vi "PicoErrorString.vi"(4 "error in":errorcluster) -> (0 "[user-defined descriptions]":string[](array[string]), 1 "String":string, 3 "[user-defined codes]":u32[](array[numeric])=[5001, 5002, 5003, 5004, 5005, 5006, 5007, 5008, 5009, 5010, 5011, 5012, 5013, 5014, 5015, 5016, 5017, 5018, 5019, 5020, 5021, 5022, 5023, 5024, 5025, 5026, 5027, 5028, 5029, 5030, 5031, 5032, 5033, 5034, 5035, 5036, 5037, 5038, 5039, 5040, 5041, 5042, 5043, 5044, 5045, 5046, 5047, 5048, 5049, 5050, 5051, 5052, 5053, 5054, 5055, 5056, 5057, 5058, 5059, 5060, 5061, 5063, 5064, 5065, 5066, 5067, 5068, 5069, 5070, 5071, 5072, 5073, 5074, 5075, 5076, 5077, 5078, 5079, 5080, 5081, 5082, 5083, 5084, 5086, 5087, 5088, 5089, 5259, 5260, 5261, 5262, 5263, 5264, 5265, 5266, 5267, 5268, 5269, 5270, 5271, 5272, 5273, 5274, 5275, 5276, 5277, 5278, 5279, 5280, 5281, 5282, 5283, 5284, 5285, 5286, 5287, 5288, 5289, 5290, 5291, 5292, 5293, 5294, 5295, 5296, 5297, 5298, 5299, 5300, 5301, 5302, 5303, 5304, 5305, 5306, 5307, 5308, 5309, 5310, 5311, 5312, 5313, 5314, 5315, 5316, 5317, 5318, 5319, 5320, 5321, 5090, 5091, 5092, 5093, 5094, 5095, 5096, 5097, 5322, 5323, 5324, 5325, 5326, 5327, 5328, 5329, 5330, 5331, 5332, 5333, 5334, 5335, 5336, 5337, 5338, 5339, 5340, 5341, 5342, 5343, 16782216, 268440456, 268440457, 268440458, 268440459, 268440460, 268440461, 268440462, 268440463, 268440464, 285217672])   [LabVIEW 2020]
doc: "This VI takes an error cluster and if an error has occurred, displays a message box indicating the source of the error and the status code returned by the driver."
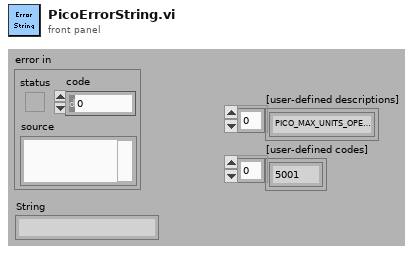
[diagram p1: front panel]
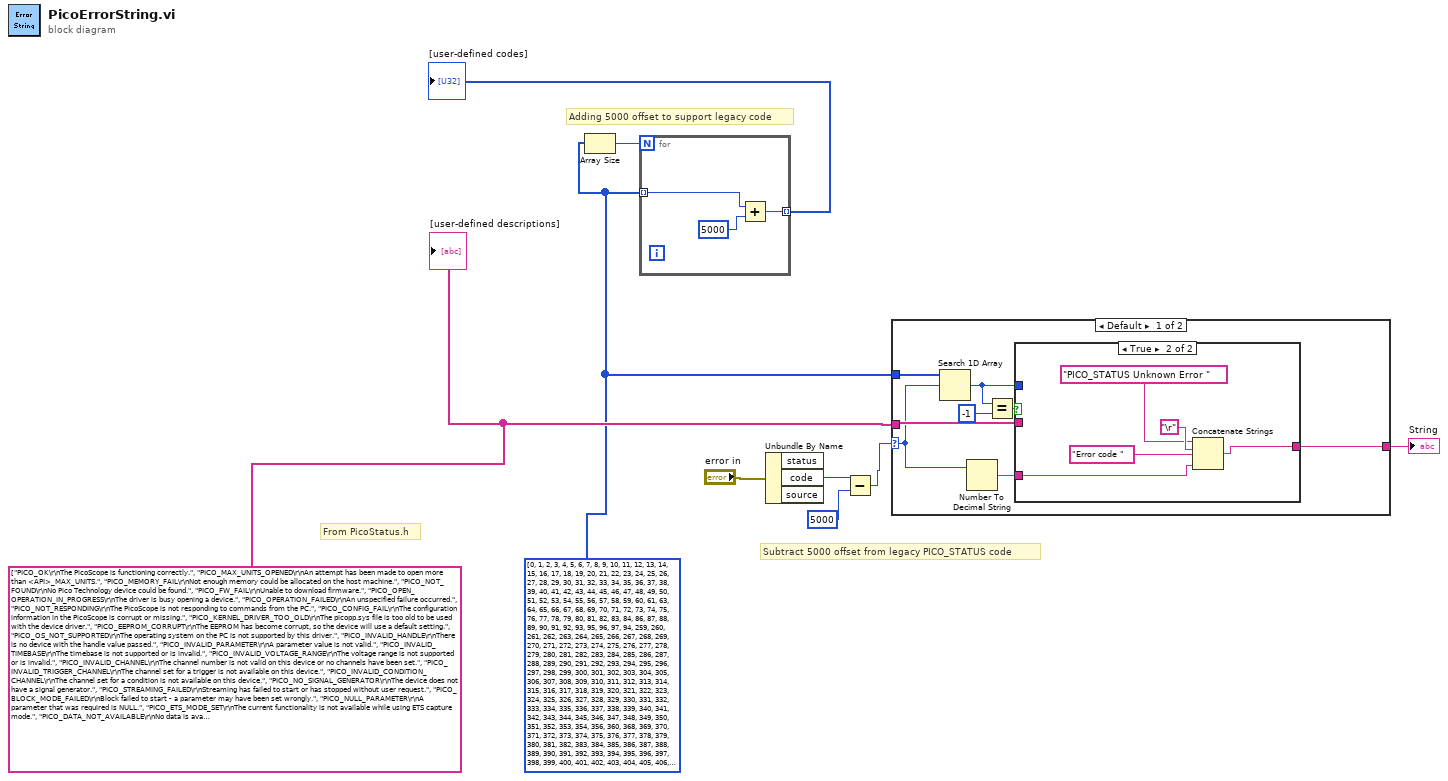
[diagram p0: block diagram]
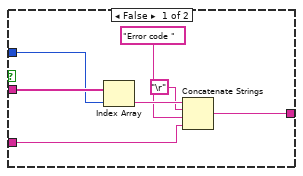
[diagram p2: hidden frame]
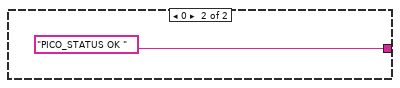
[diagram p3: hidden frame]
diagram:
  w1 = u32[] [0, 1, 2, 3, 4, 5, 6, 7, 8, 9, 10, 11, 12, 13, 14, 15, 16, 17, 18, 19, 20, 21, 22, 23, 24, 25, 26, 27, 28, 29, 30, 31, 32, 33, 34, 35, 36, 37, 38, 39, 40, 41, 42, 43, 44, 45, 46, 47, 48, 49, 50, 51, 52, 53, 54, 55, 56, 57, 58, 59, 60, 61, 63, 64, 65, 66, 67, 68, 69, 70, 71, 72, 73, 74, 75, 76, 77, 78, 79, 80, 81, 82, 83, 84, 86, 87, 88, 89, 90, 91, 92, 93, 95, 96, 97, 94, 259, 260, 261, 262, 263, 264, 265, 266, 267, 268, 269, 270, 271, 272, 273, 274, 275, 276, 277, 278, 279, 280, 281, 282, 283, 284, 285, 286, 287, 288, 289, 290, 291, 292, 293, 294, 295, 296, 297, 298, 299, 300, 301, 302, 303, 304, 305, 306, 307, 308, 309, 310, 311, 312, 313, 314, 315, 316, 317, 318, 319, 320, 321, 322, 323, 324, 325, 326, 327, 328, 329, 330, 331, 332, 333, 334, 335, 336, 337, 338, 339, 340, 341, 342, 343, 344, 345, 346, 347, 348, 349, 350, 351, 352, 353, 354, 356, 360, 368, 369, 370, 371, 372, 373, 374, 375, 376, 377, 378, 379, 380, 381, 382, 383, 384, 385, 386, 387, 388, 389, 390, 391, 392, 393, 394, 395, 396, 397, 398, 399, 400, 401, 402, 403, 404, 405, 406, 407, 408, 409, 410, 411, 412, 413, 512, 513, 514, 515, 516, 521, 522, 523, 524, 525, 526, 528, 529, 530, 531, 768, 769, 770, 4096, 4097, 8192, 8193, 8194, 8195, 8196, 8197, 8198, 8199, 8200, 8203, 8204, 8205, 8206, 8207, 8208, 8209, 8210, 8211, 8212, 8213, 8214, 8215, 8216, 8217, 12288, 12289, 12290, 12291, 12292, 12293, 12294, 12295, 12296, 12297, 12298, 12299, 16384, 20480, 20481, 20482, 20483, 20484, 20485, 20496, 24576, 24577, 24578, 28672, 28673, 28674, 16777216, 33554433, 33554434, 33554436, 33554440, 33554688, 35651584, 35651585, 35651586, 35651587, 35651588, 35651589, 35651590, 35651591, 50331664, 50331665, 50331666, 50331667, 50331668, 50331669, 50331680, 50331681, 50331682, 50331683, 50331684, 50331685, 50331686, 50331687, 50331696, 50331697, 50331698, 50331699, 50331700, 50331701, 50331702, 50331703, 50331704, 50331705, 50331712, 50335744, 50343937, 50343938, 50343939, 50345984, 50348032, 50348033, 50348034, 50348035, 50348036, 50348037, 50348038, 50348039, 50348040, 50348041, 50364416, 50364417, 50339840, 268435456, 268435457, 268435458, 268435459, 268435460, 268435461, 268435462, 268435463, 268435464, 268435472, 285212672, 536870912, 536870913, 536870914, 536870915, 536870916, 536870917, 536870918, 536870919, 536870920, 536870921] ("PICO_STATUS codes")
  w2 = string[] ["PICO_OK\r\nThe PicoScope is functioning correctly.", "PICO_MAX_UNITS_OPENED\r\nAn attempt has been made to open more than <API>_MAX_UNITS.", "PICO_MEMORY_FAIL\r\nNot enough memory could be allocated on the host machine.", "PICO_NOT_FOUND\r\nNo Pico Technology device could be found.", "PICO_FW_FAIL\r\nUnable to download firmware.", "PICO_OPEN_OPERATION_IN_PROGRESS\r\nThe driver is busy opening a device.", "PICO_OPERATION_FAILED\r\nAn unspecified failure occurred.", "PICO_NOT_RESPONDING\r\nThe PicoScope is not responding to commands from the PC.", "PICO_CONFIG_FAIL\r\nThe configuration information in the PicoScope is corrupt or missing.", "PICO_KERNEL_DRIVER_TOO_OLD\r\nThe picopp.sys file is too old to be used with the device driver.", "PICO_EEPROM_CORRUPT\r\nThe EEPROM has become corrupt, so the device will use a default setting.", "PICO_OS_NOT_SUPPORTED\r\nThe operating system on the PC is not supported by this driver.", "PICO_INVALID_HANDLE\r\nThere is no device with the handle value passed.", "PICO_INVALID_PARAMETER\r\nA parameter value is not valid.", "PICO_INVALID_TIMEBASE\r\nThe timebase is not supported or is invalid.", "PICO_INVALID_VOLTAGE_RANGE\r\nThe voltage range is not supported or is invalid.", "PICO_INVALID_CHANNEL\r\nThe channel number is not valid on this device or no channels have been set.", "PICO_INVALID_TRIGGER_CHANNEL\r\nThe channel set for a trigger is not available on this device.", "PICO_INVALID_CONDITION_CHANNEL\r\nThe channel set for a condition is not available on this device.", "PICO_NO_SIGNAL_GENERATOR\r\nThe device does not have a signal generator.", "PICO_STREAMING_FAILED\r\nStreaming has failed to start or has stopped without user request.", "PICO_BLOCK_MODE_FAILED\r\nBlock failed to start - a parameter may have been set wrongly.", "PICO_NULL_PARAMETER\r\nA parameter that was required is NULL.", "PICO_ETS_MODE_SET\r\nThe current functionality is not available while using ETS capture mode.", "PICO_DATA_NOT_AVAILABLE\r\nNo data is available from a run block call.", "PICO_STRING_BUFFER_TO_SMALL\r\nThe buffer passed for the information was too small.", "PICO_ETS_NOT_SUPPORTED\r\nETS is not supported on this device.", "PICO_AUTO_TRIGGER_TIME_TO_SHORT\r\nThe auto trigger time is less than the time it will take to collect the pre-trigger data.", "PICO_BUFFER_STALL\r\nThe collection of data has stalled as unread data would be overwritten.", "PICO_TOO_MANY_SAMPLES\r\nNumber of samples requested is more than available in the current memory segment.", "PICO_TOO_MANY_SEGMENTS\r\nNot possible to create number of segments requested.", "PICO_PULSE_WIDTH_QUALIFIER\r\nA null pointer has been passed in the trigger function or one of the parameters is out of range.", "PICO_DELAY\r\nOne or more of the hold-off parameters are out of range.", "PICO_SOURCE_DETAILS\r\nOne or more of the source details are incorrect.", "PICO_CONDITIONS\r\nOne or more of the conditions are incorrect.", "PICO_USER_CALLBACK\r\nThe driver's thread is currently in the <API>Ready callback\r\nfunction and therefore the action cannot be carried out.", "PICO_DEVICE_SAMPLING\r\nAn attempt is being made to get stored data while streaming.\r\nEither stop streaming by calling <API>Stop, or use <API>GetStreamingLatestValues.", "PICO_NO_SAMPLES_AVAILABLE\r\nData is unavailable because a run has not been completed.", "PICO_SEGMENT_OUT_OF_RANGE\r\nThe memory segment index is out of range.", "PICO_BUSY\r\nThe device is busy so data cannot be returned yet.", "PICO_STARTINDEX_INVALID\r\nThe start time to get stored data is out of range.", "PICO_INVALID_INFO\r\nThe information number requested is not a valid number.", "PICO_INFO_UNAVAILABLE\r\nThe handle is invalid so no information is available about the device.\r\nOnly PICO_DRIVER_VERSION is available.", "PICO_INVALID_SAMPLE_INTERVAL\r\nThe sample interval selected for streaming is out of range.", "PICO_TRIGGER_ERROR\r\nETS is set but no trigger has been set. A trigger setting is required for ETS.", "PICO_MEMORY\r\nDriver cannot allocate memory.", "PICO_SIG_GEN_PARAM\r\nIncorrect parameter passed to the signal generator.", "PICO_SHOTS_SWEEPS_WARNING\r\nConflict between the shots and sweeps parameters sent to the signal generator.", "PICO_SIGGEN_TRIGGER_SOURCE\r\nA software trigger has been sent but the trigger source is not a software trigger.", "PICO_AUX_OUTPUT_CONFLICT\r\nAn <API>SetTrigger call has found a conflict between the trigger source and the AUX output enable.", "PICO_AUX_OUTPUT_ETS_CONFLICT\r\nETS mode is being used and AUX is set as an input.", "PICO_WARNING_EXT_THRESHOLD_CONFLICT\r\nAttempt to set different EXT input thresholds set for signal generator and oscilloscope trigger.", "PICO_WARNING_AUX_OUTPUT_CONFLICT\r\nAn <API>SetTrigger... function has set AUX as an output and the signal generator is using it as a trigger.", "PICO_SIGGEN_OUTPUT_OVER_VOLTAGE\r\nThe combined peak-to-peak voltage and the analog offset voltage exceed the maximum voltage the signal generator can produce.", "PICO_DELAY_NULL\r\nNULL pointer passed as delay parameter.", "PICO_INVALID_BUFFER\r\nThe buffers for overview data have not been set while streaming.", "PICO_SIGGEN_OFFSET_VOLTAGE\r\nThe analog offset voltage is out of range.", "PICO_SIGGEN_PK_TO_PK\r\nThe analog peak-to-peak voltage is out of range.", "PICO_CANCELLED\r\nA block collection has been cancelled.", "PICO_SEGMENT_NOT_USED\r\nThe segment index is not currently being used.", "PICO_INVALID_CALL\r\nThe wrong GetValues function has been called for the collection mode in use.", "PICO_GET_VALUES_INTERRUPTED", "PICO_NOT_USED\r\nThe function is not available.", "PICO_INVALID_SAMPLERATIO\r\nThe aggregation ratio requested is out of range.", "PICO_INVALID_STATE\r\nDevice is in an invalid state.", "PICO_NOT_ENOUGH_SEGMENTS\r\nThe number of segments allocated is fewer than the number of captures requested.", "PICO_DRIVER_FUNCTION\r\nA driver function has already been called and not yet finished.\r\nOnly one call to the driver can be made at any one time.", "PICO_RESERVED\r\nNot used.", "PICO_INVALID_COUPLING\r\nAn invalid coupling type was specified in <API>SetChannel.", "PICO_BUFFERS_NOT_SET\r\nAn attempt was made to get data before a data buffer was defined.", "PICO_RATIO_MODE_NOT_SUPPORTED\r\nThe selected downsampling mode (used for data reduction) is not allowed.", "PICO_RAPID_NOT_SUPPORT_AGGREGATION\r\nAggregation was requested in rapid block mode.", "PICO_INVALID_TRIGGER_PROPERTY\r\nAn invalid parameter was passed to <API>SetTriggerChannelProperties(V2).", "PICO_INTERFACE_NOT_CONNECTED\r\nThe driver was unable to contact the oscilloscope.", "PICO_RESISTANCE_AND_PROBE_NOT_ALLOWED\r\nResistance-measuring mode is not allowed in conjunction with the specified probe.", "PICO_POWER_FAILED\r\nThe device was unexpectedly powered down.", "PICO_SIGGEN_WAVEFORM_SETUP_FAILED\r\nA problem occurred in <API>SetSigGenBuiltIn or <API>SetSigGenArbitrary.", "PICO_FPGA_FAIL\r\nFPGA not successfully set up.", "PICO_POWER_MANAGER", "PICO_INVALID_ANALOGUE_OFFSET\r\nAn impossible analog offset value was specified in <API>SetChannel.", "PICO_PLL_LOCK_FAILED\r\nThere is an error within the device hardware.", "PICO_ANALOG_BOARD\r\nThere is an error within the device hardware.", "PICO_CONFIG_FAIL_AWG\r\nUnable to configure the signal generator.", "PICO_INITIALISE_FPGA\r\nThe FPGA cannot be initialized, so unit cannot be opened.", "PICO_EXTERNAL_FREQUENCY_INVALID\r\nThe frequency for the external clock is not within 15% of the nominal value.", "PICO_CLOCK_CHANGE_ERROR\r\nThe FPGA could not lock the clock signal.", "PICO_TRIGGER_AND_EXTERNAL_CLOCK_CLASH\r\nYou are trying to configure the AUX input as both a trigger and a reference clock.", "PICO_PWQ_AND_EXTERNAL_CLOCK_CLASH\r\nYou are trying to configure the AUX input as both a pulse width qualifier and a reference clock.", "PICO_UNABLE_TO_OPEN_SCALING_FILE\r\nThe requested scaling file cannot be opened.", "PICO_MEMORY_CLOCK_FREQUENCY\r\nThe frequency of the memory is reporting incorrectly.", "PICO_I2C_NOT_RESPONDING\r\nThe I2C that is being actioned is not responding to requests.", "PICO_NO_CAPTURES_AVAILABLE\r\nThere are no captures available and therefore no data can be returned.", "PICO_TOO_MANY_TRIGGER_CHANNELS_IN_USE\r\nThe number of trigger channels is greater than 4,\r\nexcept for a PicoScope 4824 where 8 channels are allowed for rising/falling/rising_or_falling trigger directions.", "PICO_INVALID_TRIGGER_DIRECTION\r\nIf you have specified a trigger direction which is not allowed, for example specifying PICO_ABOVE\r\nwithout another condition which crosses a threshold on another channel.", "PICO_INVALID_TRIGGER_STATES\r\nWhen more than 4 trigger channels are set and their trigger condition states are not <API>_CONDITION_TRUE.", "PICO_NOT_USED_IN_THIS_CAPTURE_MODE\r\nThe capture mode the device is currently running in does not support the current request.", "PICO_GET_DATA_ACTIVE", "PICO_IP_NETWORKEDCodes 104 to 10B are used by the PT104 (USB) when connected via the Network Socket.\r\nCodes 104 to 10B are used by the PT104 (USB) when connected via the Network Socket.\r\nThe device is currently connected via the IP Network socket and thus the call made is not supported.", "PICO_INVALID_IP_ADDRESS\r\nAn incorrect IP address has been passed to the driver.", "PICO_IPSOCKET_FAILED\r\nThe IP socket has failed.", "PICO_IPSOCKET_TIMEDOUT\r\nThe IP socket has timed out.", "PICO_SETTINGS_FAILED\r\nFailed to apply the requested settings.", "PICO_NETWORK_FAILED\r\nThe network connection has failed.", "PICO_WS2_32_DLL_NOT_LOADED\r\nUnable to load the WS2 DLL.", "PICO_INVALID_IP_PORT\r\nThe specified IP port is invalid.", "PICO_COUPLING_NOT_SUPPORTED\r\nThe type of coupling requested is not supported on the opened device.", "PICO_BANDWIDTH_NOT_SUPPORTED\r\nBandwidth limiting is not supported on the opened device.", "PICO_INVALID_BANDWIDTH\r\nThe value requested for the bandwidth limit is out of range.", "PICO_AWG_NOT_SUPPORTED\r\nThe arbitrary waveform generator is not supported by the opened device.", "PICO_ETS_NOT_RUNNING\r\nData has been requested with ETS mode set but run block has not been called,\r\nor stop has been called.", "PICO_SIG_GEN_WHITENOISE_NOT_SUPPORTED\r\nWhite noise output is not supported on the opened device.", "PICO_SIG_GEN_WAVETYPE_NOT_SUPPORTED\r\nThe wave type requested is not supported by the opened device.", "PICO_INVALID_DIGITAL_PORT\r\nThe requested digital port number is out of range (MSOs only).", "PICO_INVALID_DIGITAL_CHANNEL\r\nThe digital channel is not in the range <API>_DIGITAL_CHANNEL0 to\r\n<API>_DIGITAL_CHANNEL15, the digital channels that are supported.", "PICO_INVALID_DIGITAL_TRIGGER_DIRECTION\r\nThe digital trigger direction is not a valid trigger direction and should be equal\r\nin value to one of the <API>_DIGITAL_DIRECTION enumerations.", "PICO_SIG_GEN_PRBS_NOT_SUPPORTED\r\nSignal generator does not generate pseudo-random binary sequence.", "PICO_ETS_NOT_AVAILABLE_WITH_LOGIC_CHANNELS\r\nWhen a digital port is enabled, ETS sample mode is not available for use.", "PICO_WARNING_REPEAT_VALUE\r\nThere has been no new sample taken, this value has already been returned previously.", "PICO_POWER_SUPPLY_CONNECTED\r\nThe DC power supply is connected.", "PICO_POWER_SUPPLY_NOT_CONNECTED\r\nThe DC power supply is not connected.\r\nFor many 4+ Channel devices this will mean a restricted feature set is offered e.g. for a 4 channel device - C and D are usually disabled.\r\nCheck the respective API programmers guide of your device for the full details.", "PICO_POWER_SUPPLY_REQUEST_INVALID\r\nIncorrect power mode passed for current power source.", "PICO_POWER_SUPPLY_UNDERVOLTAGE\r\nThe supply voltage from the USB source is too low.", "PICO_CAPTURING_DATA\r\nThe oscilloscope is in the process of capturing data.", "PICO_USB3_0_DEVICE_NON_USB3_0_PORT\r\nA USB 3.0 device is connected to a non-USB 3.0 port.", "PICO_NOT_SUPPORTED_BY_THIS_DEVICE\r\nA function has been called that is not supported by the current device.", "PICO_INVALID_DEVICE_RESOLUTION\r\nThe device resolution is invalid (out of range).", "PICO_INVALID_NUMBER_CHANNELS_FOR_RESOLUTION\r\nThe number of channels that can be enabled is limited in 15 and 16-bit modes.\r\n(Flexible Resolution Oscilloscopes only)", "PICO_CHANNEL_DISABLED_DUE_TO_USB_POWERED\r\nUSB power not sufficient for all requested channels.", "PICO_SIGGEN_DC_VOLTAGE_NOT_CONFIGURABLE\r\nThe signal generator does not have a configurable DC offset.", "PICO_NO_TRIGGER_ENABLED_FOR_TRIGGER_IN_PRE_TRIG\r\nAn attempt has been made to define pre-trigger delay without first enabling a trigger.", "PICO_TRIGGER_WITHIN_PRE_TRIG_NOT_ARMED\r\nAn attempt has been made to define pre-trigger delay without first arming a trigger.", "PICO_TRIGGER_WITHIN_PRE_NOT_ALLOWED_WITH_DELAY\r\nPre-trigger delay and post-trigger delay cannot be used at the same time.", "PICO_TRIGGER_INDEX_UNAVAILABLE\r\nThe array index points to a nonexistent trigger.", "PICO_AWG_CLOCK_FREQUENCY", "PICO_TOO_MANY_CHANNELS_IN_USE\r\nThere are more than 4 analog channels with a trigger condition set.", "PICO_NULL_CONDITIONS\r\nThe condition parameter is a null pointer.", "PICO_DUPLICATE_CONDITION_SOURCE\r\nThere is more than one condition pertaining to the same channel.", "PICO_INVALID_CONDITION_INFO\r\nThe parameter relating to condition information is out of range.", "PICO_SETTINGS_READ_FAILED\r\nReading the meta data has failed.", "PICO_SETTINGS_WRITE_FAILED\r\nWriting the meta data has failed.", "PICO_ARGUMENT_OUT_OF_RANGE\r\nA parameter has a value out of the expected range.", "PICO_HARDWARE_VERSION_NOT_SUPPORTED\r\nThe driver does not support the hardware variant connected.", "PICO_DIGITAL_HARDWARE_VERSION_NOT_SUPPORTED\r\nThe driver does not support the digital hardware variant connected.", "PICO_ANALOGUE_HARDWARE_VERSION_NOT_SUPPORTED\r\nThe driver does not support the analog hardware variant connected.", "PICO_UNABLE_TO_CONVERT_TO_RESISTANCE\r\nConverting a channel's ADC value to resistance has failed.", "PICO_DUPLICATED_CHANNEL\r\nThe channel is listed more than once in the function call.", "PICO_INVALID_RESISTANCE_CONVERSION\r\nThe range cannot have resistance conversion applied.", "PICO_INVALID_VALUE_IN_MAX_BUFFER\r\nAn invalid value is in the max buffer.", "PICO_INVALID_VALUE_IN_MIN_BUFFER\r\nAn invalid value is in the min buffer.", "PICO_SIGGEN_FREQUENCY_OUT_OF_RANGE\r\nWhen calculating the frequency for phase conversion,\r\nthe frequency is greater than that supported by the current variant.", "PICO_EEPROM2_CORRUPT\r\nThe device's EEPROM is corrupt. Contact Pico Technology support: https://www.picotech.com/tech-support.", "PICO_EEPROM2_FAIL\r\nThe EEPROM has failed.", "PICO_SERIAL_BUFFER_TOO_SMALL\r\nThe serial buffer is too small for the required information.", "PICO_SIGGEN_TRIGGER_AND_EXTERNAL_CLOCK_CLASH\r\nThe signal generator trigger and the external clock have both been set.\r\nThis is not allowed.", "PICO_WARNING_SIGGEN_AUXIO_TRIGGER_DISABLED\r\nThe AUX trigger was enabled and the external clock has been enabled,\r\nso the AUX has been automatically disabled.", "PICO_SIGGEN_GATING_AUXIO_NOT_AVAILABLE\r\nThe AUX I/O was set as a scope trigger and is now being set as a signal generator\r\ngating trigger. This is not allowed.", "PICO_SIGGEN_GATING_AUXIO_ENABLED\r\nThe AUX I/O was set by the signal generator as a gating trigger and is now being set\r\nas a scope trigger. This is not allowed.", "PICO_RESOURCE_ERROR\r\nA resource has failed to initialise.", "PICO_TEMPERATURE_TYPE_INVALID\r\nThe temperature type is out of range.", "PICO_TEMPERATURE_TYPE_NOT_SUPPORTED\r\nA requested temperature type is not supported on this device.", "PICO_TIMEOUT\r\nA read/write to the device has timed out.", "PICO_DEVICE_NOT_FUNCTIONING\r\nThe device cannot be connected correctly.", "PICO_INTERNAL_ERROR\r\nThe driver has experienced an unknown error and is unable to recover from this error.", "PICO_MULTIPLE_DEVICES_FOUND\r\nUsed when opening units via IP and more than multiple units have the same IP address.", "PICO_WARNING_NUMBER_OF_SEGMENTS_REDUCED", "PICO_CAL_PINS_STATES\r\nThe calibration pin states argument is out of range.", "PICO_CAL_PINS_FREQUENCY\r\nThe calibration pin frequency argument is out of range.", "PICO_CAL_PINS_AMPLITUDE\r\nThe calibration pin amplitude argument is out of range.", "PICO_CAL_PINS_WAVETYPE\r\nThe calibration pin wavetype argument is out of range.", "PICO_CAL_PINS_OFFSET\r\nThe calibration pin offset argument is out of range.", "PICO_PROBE_FAULT\r\nThe probe's identity has a problem.", "PICO_PROBE_IDENTITY_UNKNOWN\r\nThe probe has not been identified.", "PICO_PROBE_POWER_DC_POWER_SUPPLY_REQUIRED\r\nEnabling the probe would cause the device to exceed the allowable current limit.", "PICO_PROBE_NOT_POWERED_WITH_DC_POWER_SUPPLY\r\nThe DC power supply is connected; enabling the probe would cause the device to exceed the\r\nallowable current limit.", "PICO_PROBE_CONFIG_FAILURE\r\nFailed to complete probe configuration.", "PICO_PROBE_INTERACTION_CALLBACK\r\nFailed to set the callback function, as currently in current callback function.", "PICO_UNKNOWN_INTELLIGENT_PROBE\r\nThe probe has been verified but not known on this driver.", "PICO_INTELLIGENT_PROBE_CORRUPT\r\nThe intelligent probe cannot be verified.", "PICO_PROBE_COLLECTION_NOT_STARTED\r\nThe callback is null, probe collection will only start when\r\nfirst callback is a none null pointer.", "PICO_PROBE_POWER_CONSUMPTION_EXCEEDED\r\nThe current drawn by the probe(s) has exceeded the allowed limit.", "PICO_WARNING_PROBE_CHANNEL_OUT_OF_SYNC\r\nThe channel range limits have changed due to connecting or disconnecting a probe\r\nthe channel has been enabled.", "PICO_ENDPOINT_MISSING", "PICO_UNKNOWN_ENDPOINT_REQUEST", "PICO_ADC_TYPE_ERROR\r\nThe ADC on board the device has not been correctly identified.", "PICO_FPGA2_FAILED", "PICO_FPGA2_DEVICE_STATUS", "PICO_ENABLE_PROGRAM_FPGA2_FAILED", "PICO_NO_CHANNELS_OR_PORTS_ENABLED", "PICO_INVALID_RATIO_MODE", "PICO_READS_NOT_SUPPORTED_IN_CURRENT_CAPTURE_MODE", "PICO_TRIGGER_READ_SELECTION_CHECK_FAILED\r\nThese selection tests can be masked together to show that mode than one read selection has failed the tests,\r\ntherefore theses error codes cover 0x00000161UL to 0x0000016FUL.", "PICO_DATA_READ1_SELECTION_CHECK_FAILED", "PICO_DATA_READ2_SELECTION_CHECK_FAILED", "PICO_DATA_READ3_SELECTION_CHECK_FAILED", "PICO_READ_SELECTION_OUT_OF_RANGE\r\nThe requested read is not one of the reads available in enPicoReadSelection.", "PICO_MULTIPLE_RATIO_MODES\r\nThe downsample ratio options cannot be combined together for this request.", "PICO_NO_SAMPLES_READ\r\nThe enPicoReadSelection request has no samples available.", "PICO_RATIO_MODE_NOT_REQUESTED\r\nThe enPicoReadSelection did not include one of the downsample ratios now requested.", "PICO_NO_USER_READ_REQUESTS_SET\r\nNo read requests have been made.", "PICO_ZERO_SAMPLES_INVALID\r\nThe parameter for <number of values> cannot be zero.", "PICO_ANALOGUE_HARDWARE_MISSING\r\nThe analog hardware cannot be identified; contact Pico Technology Technical Support.", "PICO_ANALOGUE_HARDWARE_PINS\r\nSetting of the analog hardware pins failed.", "PICO_ANALOGUE_HARDWARE_SMPS_FAULT\r\nAn SMPS fault has occurred.", "PICO_DIGITAL_ANALOGUE_HARDWARE_CONFLICT\r\nThere appears to be a conflict between the expected and actual hardware in the device; contact Pico Technology Technical Support.", "PICO_RATIO_MODE_BUFFER_NOT_SET\r\nOne or more of the enPicoRatioMode requested do not have a data buffer set.", "PICO_RESOLUTION_NOT_SUPPORTED_BY_VARIANT\r\nThe resolution is valid but not supported by the opened device.", "PICO_THRESHOLD_OUT_OF_RANGE\r\nThe requested trigger threshold is out of range for the current device resolution.", "PICO_INVALID_SIMPLE_TRIGGER_DIRECTION\r\nThe simple trigger only supports upper edge direction options.", "PICO_AUX_NOT_SUPPORTED\r\nThe aux trigger is not supported on this variant.", "PICO_NULL_DIRECTIONS\r\nThe trigger directions pointer may not be null.", "PICO_NULL_CHANNEL_PROPERTIES\r\nThe trigger channel properties pointer may not be null.", "PICO_TRIGGER_CHANNEL_NOT_ENABLED\r\nA trigger is set on a channel that has not been enabled.", "PICO_CONDITION_HAS_NO_TRIGGER_PROPERTY\r\nA trigger condition has been set but a trigger property not set.", "PICO_RATIO_MODE_TRIGGER_MASKING_INVALID\r\nWhen requesting trigger data, this option can only be combined with the segment header ratio mode flag.", "PICO_TRIGGER_DATA_REQUIRES_MIN_BUFFER_SIZE_OF_40_SAMPLES\r\nThe trigger data buffer must be 40 or more samples in size.", "PICO_NO_OF_CAPTURES_OUT_OF_RANGE\r\nThe number of requested waveforms is greater than the number of memory segments allocated.", "PICO_RATIO_MODE_SEGMENT_HEADER_DOES_NOT_REQUIRE_BUFFERS\r\nWhen requesting segment header information, the segment header does not require a data buffer,\r\nto get the segment information use GetTriggerInfo.", "PICO_FOR_SEGMENT_HEADER_USE_GETTRIGGERINFO\r\nUse GetTriggerInfo to retrieve the segment header information.", "PICO_READ_NOT_SET\r\nA read request has not been set.", "PICO_ADC_SETTING_MISMATCH\r\nThe expected and actual states of the ADCs do not match.", "PICO_DATATYPE_INVALID\r\nThe requested data type is not one of the enPicoDataType listed.", "PICO_RATIO_MODE_DOES_NOT_SUPPORT_DATATYPE\r\nThe down sample ratio mode requested does not support the enPicoDataType option chosen.", "PICO_CHANNEL_COMBINATION_NOT_VALID_IN_THIS_RESOLUTION\r\nThe channel combination is not valid for the resolution.", "PICO_USE_8BIT_RESOLUTION", "PICO_AGGREGATE_BUFFERS_SAME_POINTER\r\nThe buffer for minimum data values and maximum data values are the same buffers.", "PICO_OVERLAPPED_READ_VALUES_OUT_OF_RANGE\r\nThe read request number of samples requested for an overlapped operation are more\r\nthan the total number of samples to capture.", "PICO_OVERLAPPED_READ_SEGMENTS_OUT_OF_RANGE\r\nThe overlapped read request has more segments specified than segments allocated.", "PICO_CHANNELFLAGSCOMBINATIONS_ARRAY_SIZE_TOO_SMALL\r\nThe number of channel combinations available are greater than the array size received.", "PICO_CAPTURES_EXCEEDS_NO_OF_SUPPORTED_SEGMENTS\r\nThe number of captures is larger than the maximum number of segments allowed for the device variant.", "PICO_TIME_UNITS_OUT_OF_RANGE\r\nThe time unit requested is not one of the listed enPicoTimeUnits.", "PICO_NO_SAMPLES_REQUESTED\r\nThe number of samples parameter may not be zero.", "PICO_INVALID_ACTION\r\nThe action requested is not listed in enPicoAction.", "PICO_NO_OF_SAMPLES_NEED_TO_BE_EQUAL_WHEN_ADDING_BUFFERS\r\nWhen adding buffers for the same read request the buffers for all ratio mode requests have to be the same size.", "PICO_WAITING_FOR_DATA_BUFFERS\r\nThe data is being processed but there is no empty data buffers available, a new data buffer needs to be set sent to the driver\r\nso that the data can be processed.", "PICO_STREAMING_ONLY_SUPPORTS_ONE_READ\r\nwhen streaming data, only one read option is available.", "PICO_CLEAR_DATA_BUFFER_INVALID\r\nA clear read request is not one of the enPicoAction listed.", "PICO_INVALID_ACTION_FLAGS_COMBINATION\r\nThe combination of action flags are not allowed.", "PICO_BOTH_MIN_AND_MAX_NULL_BUFFERS_CANNOT_BE_ADDED\r\nPICO_ADD request has been made but both data buffers are set to null and so there is nowhere to put the data.", "PICO_CONFLICT_IN_SET_DATA_BUFFERS_CALL_REMOVE_DATA_BUFFER_TO_RESET\r\nA conflict between the data buffers being set has occurred. Please use the PICO_CLEAR_ALL action to reset.", "PICO_REMOVING_DATA_BUFFER_ENTRIES_NOT_ALLOWED_WHILE_DATA_PROCESSING\r\nWhile processing data, buffers cannot be removed from the data buffers list.", "PICO_CYUSB_REQUEST_FAILED\r\nAn USB request has failed.", "PICO_STREAMING_DATA_REQUIRED\r\nA request has been made to retrieve the latest streaming data, but with either a null pointer or an array size set to zero.", "PICO_INVALID_NUMBER_OF_SAMPLES\r\nA buffer being set has a length that is invalid (ie less than zero).", "PICO_INVALID_DISTRIBUTION\r\nThe distribution size may not be zero.", "PICO_BUFFER_LENGTH_GREATER_THAN_INT32_T\r\nThe buffer length in bytes is greater than a 4-byte word.", "PICO_PLL_MUX_OUT_FAILED\r\nThe PLL has failed.", "PICO_ONE_PULSE_WIDTH_DIRECTION_ALLOWED\r\nPulse width only supports one direction.", "PICO_EXTERNAL_TRIGGER_NOT_SUPPORTED\r\nThere is no external trigger available on the device specified by the handle.", "PICO_NO_TRIGGER_CONDITIONS_SET\r\nThe condition parameter is a null pointer.", "PICO_NO_OF_CHANNEL_TRIGGER_PROPERTIES_OUT_OF_RANGE\r\nThe number of trigger channel properties it outside the allowed range (is less than zero).", "PICO_PROBE_COMPONENT_ERROR\r\nA probe has been plugged into a channel, but can not be identified correctly.", "PICO_INVALID_TRIGGER_CHANNEL_FOR_ETS\r\nThe requested channel for ETS triggering is not supported.", "PICO_NOT_AVAILABLE_WHEN_STREAMING_IS_RUNNING\r\nWhile the device is streaming the get values method is not available", "PICO_INVALID_TRIGGER_WITHIN_PRE_TRIGGER_STATE\r\nthe requested state is not one of the enSharedTriggerWithinPreTrigger values", "PICO_ZERO_NUMBER_OF_CAPTURES_INVALID\r\nthe number of captures have to be greater than zero", "PICO_TRIGGER_DELAY_OUT_OF_RANGE\r\nthe trigger delay is greater than supported by the hardware", "PICO_INVALID_THRESHOLD_DIRECTION\r\nthe requested threshold direction is not allowed with the specified channel", "PICO_INVALID_THRESHOLD_MODE\r\nthe requested threshold mode is not allowed with the specified channel", "PICO_INVALID_VARIANT\r\nThe device variant is not supported by this current driver.", "PICO_MEMORY_MODULE_ERROR\r\nThe actual memory module does not match the expected memory module.", "PICO_PULSE_WIDTH_QUALIFIER_LOWER_UPPER_CONFILCT\r\nA null pointer has been passed in the trigger function or one of the parameters is out of range.", "PICO_PULSE_WIDTH_QUALIFIER_TYPE\r\nThe pulse width qualifier type is not one of the listed options.", "PICO_PULSE_WIDTH_QUALIFIER_DIRECTION\r\nThe pulse width qualifier direction is not one of the listed options.", "PICO_THRESHOLD_MODE_OUT_OF_RANGE\r\nThe threshold range is not one of the listed options.", "PICO_TRIGGER_AND_PULSEWIDTH_DIRECTION_IN_CONFLICT\r\nThe trigger direction and pulse width option conflict with each other.", "PICO_THRESHOLD_UPPER_LOWER_MISMATCH\r\nThe thresholds upper limits and thresholds lower limits conflict with each other.", "PICO_PULSE_WIDTH_LOWER_OUT_OF_RANGE\r\nThe pulse width lower count is out of range.", "PICO_PULSE_WIDTH_UPPER_OUT_OF_RANGE\r\nThe pulse width upper count is out of range.", "PICO_FRONT_PANEL_ERROR\r\nThe devices front panel has caused an error.", "PICO_FRONT_PANEL_MODE\r\nThe actual and expected mode of the front panel do not match.", "PICO_FRONT_PANEL_FEATURE\r\nA front panel feature is not available or failed to configure.", "PICO_NO_PULSE_WIDTH_CONDITIONS_SET\r\nWhen setting the pulse width conditions either the pointer is null or the number of conditions is set to zero.", "PICO_TRIGGER_PORT_NOT_ENABLED\r\na trigger condition exists for a port, but the port has not been enabled", "PICO_DIGITAL_DIRECTION_NOT_SET\r\na trigger condition exists for a port, but no digital channel directions have been set", "PICO_I2C_DEVICE_INVALID_READ_COMMAND", "PICO_I2C_DEVICE_INVALID_RESPONSE", "PICO_I2C_DEVICE_INVALID_WRITE_COMMAND", "PICO_I2C_DEVICE_ARGUMENT_OUT_OF_RANGE", "PICO_I2C_DEVICE_MODE\r\nThe actual and expected mode do not match.", "PICO_I2C_DEVICE_SETUP_FAILED\r\nWhile trying to configure the device, set up failed.", "PICO_I2C_DEVICE_FEATURE\r\nA feature is not available or failed to configure.", "PICO_I2C_DEVICE_VALIDATION_FAILED\r\nThe device did not pass the validation checks.", "PICO_INTERNAL_HEADER_ERROR", "PICO_FAILED_TO_WRITE_HARDWARE_FAULT\r\nThe device couldn't write the channel settings due to a hardware fault", "PICO_MSO_TOO_MANY_EDGE_TRANSITIONS_WHEN_USING_PULSE_WIDTH\r\nThe number of MSO's edge transitions being set is not supported by this device (RISING, FALLING, or RISING_OR_FALLING).", "PICO_INVALID_PROBE_LED_POSITION\r\nA probe LED position requested is not one of the available probe positions in the ProbeLedPosition enum.", "PICO_PROBE_LED_POSITION_NOT_SUPPORTED\r\nThe LED position is not supported by the selected variant.", "PICO_DUPLICATE_PROBE_CHANNEL_LED_POSITION\r\nA channel has more than one of the same LED position in the ProbeChannelLedSetting struct.", "PICO_PROBE_LED_FAILURE\r\nSetting the probes LED has failed.", "PICO_PROBE_NOT_SUPPORTED_BY_THIS_DEVICE\r\nProbe is not supported by the selected variant.", "PICO_INVALID_PROBE_NAME\r\nThe probe name is not in the list of enPicoConnectProbe enums.", "PICO_NO_PROBE_COLOUR_SETTINGS\r\nThe number of colour settings are zero or a null pointer passed to the function.", "PICO_NO_PROBE_CONNECTED_ON_REQUESTED_CHANNEL\r\nChannel has no probe connected to it.", "PICO_PROBE_DOES_NOT_REQUIRE_CALIBRATION\r\nConnected probe does not require calibration.", "PICO_PROBE_CALIBRATION_FAILED\r\nConnected probe could not be calibrated - hardware fault is a possible cause.", "PICO_PROBE_VERSION_ERROR\r\nA probe has been connected, but the version is not recognised.", "PICO_AUTO_TRIGGER_TIME_TOO_LONG\r\nThe requested trigger time is to long for the selected variant.", "PICO_MSO_POD_VALIDATION_FAILED\r\nThe MSO pod did not pass the validation checks.", "PICO_NO_MSO_POD_CONNECTED\r\nNo MSO pod found on the requested digital port.", "PICO_DIGITAL_PORT_HYSTERESIS_OUT_OF_RANGE\r\nthe digital port enum value is not in the enPicoDigitalPortHysteresis declaration", "PICO_MSO_POD_FAILED_UNIT", "PICO_ATTENUATION_FAILED\r\nThe device's EEPROM is corrupt. Contact Pico Technology support: https://www.picotech.com/tech-support.", "PICO_DC_50OHM_OVERVOLTAGE_TRIPPED\r\na channel set to the 50Ohm Path has Tripped due to the input signal", "PICO_NOT_RESPONDING_OVERHEATED\r\nStatus error for when the device has overheated.", "PICO_HARDWARE_CAPTURE_TIMEOUT\r\nwaiting for the device to capture timed out", "PICO_HARDWARE_READY_TIMEOUT\r\nwaiting for the device be ready for capture timed out", "PICO_HARDWARE_CAPTURING_CALL_STOP\r\nthe driver is performing a capture requested by RunStreaming or RunBlock\r\nto interrupt this capture call Stop on the device first", "PICO_TOO_FEW_REQUESTED_STREAMING_SAMPLES\r\nthe number of samples is less than the minimum number allowed", "PICO_STREAMING_REREAD_DATA_NOT_AVAILABLE\r\na streaming capture has been made but re-reading the data is not allowed", "PICO_STREAMING_COMBINATION_OF_RAW_DATA_AND_ONE_AGGREGATION_DATA_TYPE_ALLOWEDaverage and sum are classed as one aggregation type", "PICO_DEVICE_TIME_STAMP_RESET\r\nThe time stamp per waveform segment has been reset.", "PICO_TRIGGER_TIME_NOT_REQUESTED\r\nWhen requesting the TriggerTimeOffset the trigger time has not been set.", "PICO_TRIGGER_TIME_BUFFER_NOT_SET\r\nTrigger time buffer not set.", "PICO_TRIGGER_TIME_FAILED_TO_CALCULATE\r\nThe trigger time failed to be calculated.", "PICO_TRIGGER_WITHIN_A_PRE_TRIGGER_FAILED_TO_CALCULATE\r\nThe trigger time failed to be calculated.", "PICO_TRIGGER_TIME_STAMP_NOT_REQUESTED\r\nThe trigger time stamp was not requested.", "PICO_RATIO_MODE_TRIGGER_DATA_FOR_TIME_CALCULATION_DOES_NOT_REQUIRE_BUFFERS\r\nRATIO_MODE_TRIGGER_DATA_FOR_TIME_CALCULATION cannot have a buffer set", "PICO_RATIO_MODE_TRIGGER_DATA_FOR_TIME_CALCULATION_DOES_NOT_HAVE_BUFFERS\r\nit is not possible to set a buffer for RATIO_MODE_TRIGGER_DATA_FOR_TIME_CALCULATION therefore\r\ninformation is not available pertaining to samples", "PICO_RATIO_MODE_TRIGGER_DATA_FOR_TIME_CALCULATION_USE_GETTRIGGERINFO\r\nto get the trigger time use either GetTriggerInfo or GetTriggerTimeOffset api calls", "PICO_STREAMING_DOES_NOT_SUPPORT_TRIGGER_RATIO_MODES\r\nPICO_RATIO_MDOE_TRIGGER and RATIO_MODE_TRIGGER_DATA_FOR_TIME_CALCULATION is not supported in streaming capture", "PICO_USE_THE_TRIGGER_READ\r\nonly the PICO_TRIGGER_READ may be used to read PICO_RATIO_MODE_TRIGGER, and PICO_RATIO_MODE_TRIGGER_FOR_CALCULATION", "PICO_USE_A_DATA_READ\r\none of the PICO_DATA_READs should be used to read:\r\nPICO_RATIO_MODE_RAW\r\nPICO_RATIO_MODE_AGGREGATE\r\nPICO_RATIO_MODE_DECIMATE\r\nPICO_RATIO_MODE_AVERAGE", "PICO_TRIGGER_READ_REQUIRES_INT16_T_DATA_TYPE\r\ntrigger data always requires a PICO_INT16_T data type", "PICO_RATIO_MODE_REQUIRES_NUMBER_OF_SAMPLES_TO_BE_SET\r\na ratio mode passed to the API call requires the number of samples to be greater than zero", "PICO_SIGGEN_SETTINGS_MISMATCH\r\nAttempted to set up the signal generator with an inconsistent configuration.", "PICO_SIGGEN_SETTINGS_CHANGED_CALL_APPLY\r\nThe signal generator has been partially reconfigured and the new settings must be applied before it can be paused or restarted.", "PICO_SIGGEN_WAVETYPE_NOT_SUPPORTED\r\nThe wave type is not listed in enPicoWaveType.", "PICO_SIGGEN_TRIGGERTYPE_NOT_SUPPORTED\r\nThe trigger type is not listed in enSigGenTrigType.", "PICO_SIGGEN_TRIGGERSOURCE_NOT_SUPPORTED\r\nThe trigger source is not listed in enSigGenTrigSource.", "PICO_SIGGEN_FILTER_STATE_NOT_SUPPORTED\r\nThe filter state is not listed in enPicoSigGenFilterState.", "PICO_SIGGEN_NULL_PARAMETER\r\nThe arbitrary waveform buffer is a null pointer.", "PICO_SIGGEN_EMPTY_BUFFER_SUPPLIED\r\nThe arbitrary waveform buffer length is zero.", "PICO_SIGGEN_RANGE_NOT_SUPPLIED\r\nThe sig gen voltage offset and peak to peak have not been set.", "PICO_SIGGEN_BUFFER_NOT_SUPPLIED\r\nThe sig gen arbitrary waveform buffer not been set.", "PICO_SIGGEN_FREQUENCY_NOT_SUPPLIED\r\nThe sig gen frequency have not been set.", "PICO_SIGGEN_SWEEP_INFO_NOT_SUPPLIED\r\nThe sig gen sweep information has not been set.", "PICO_SIGGEN_TRIGGER_INFO_NOT_SUPPLIED\r\nThe sig gen trigger information has not been set.", "PICO_SIGGEN_CLOCK_FREQ_NOT_SUPPLIED\r\nThe sig gen clock frequency have not been set.", "PICO_SIGGEN_TOO_MANY_SAMPLES\r\nThe sig gen arbitrary waveform buffer length is too long.", "PICO_SIGGEN_DUTYCYCLE_OUT_OF_RANGE\r\nThe duty cycle value is out of range.", "PICO_SIGGEN_CYCLES_OUT_OF_RANGE\r\nThe number of cycles is out of range.", "PICO_SIGGEN_PRESCALE_OUT_OF_RANGE\r\nThe pre-scaler is out of range.", "PICO_SIGGEN_SWEEPTYPE_INVALID\r\nThe sweep type is not listed in enPicoSweepType.", "PICO_SIGGEN_SWEEP_WAVETYPE_MISMATCH\r\nA mismatch has occurred while checking the sweeps wave type.", "PICO_SIGGEN_INVALID_SWEEP_PARAMETERS\r\nThe sweeps or shots and trigger type are not valid when combined together.", "PICO_SIGGEN_SWEEP_PRESCALE_NOT_SUPPORTED\r\nThe sweep and prescaler are not valid when combined together.", "PICO_AWG_OVER_VOLTAGE_RANGE\r\nThe potential applied to the AWG output exceeds the maximum voltage range of the AWG.", "PICO_NOT_LOCKED_TO_REFERENCE_FREQUENCY\r\nThe reference signal cannot be locked to.", "PICO_PERMISSIONS_ERROR\r\n(Linux only.) udev rules are incorrectly configured. The user does\r\nnot have read/write permissions on the device's file descriptor.", "PICO_PORTS_WITHOUT_ANALOGUE_CHANNELS_ONLY_ALLOWED_IN_8BIT_RESOLUTION\r\nThe digital ports without analog channels are only allowed in 8-bit resolution.", "PICO_ANALOGUE_FRONTEND_MISSING", "PICO_FRONT_PANEL_MISSING", "PICO_ANALOGUE_FRONTEND_AND_FRONT_PANEL_MISSING", "PICO_DIGITAL_BOARD_HARDWARE_ERROR\r\nThe digital board has reported an error to the driver", "PICO_FIRMWARE_UPDATE_REQUIRED_TO_USE_DEVICE_WITH_THIS_DRIVER\r\nchecking if the firmware needs updating the updateRequired parameter is null", "PICO_UPDATE_REQUIRED_NULL", "PICO_FIRMWARE_UP_TO_DATE", "PICO_FLASH_FAIL", "PICO_INTERNAL_ERROR_FIRMWARE_LENGTH_INVALID", "PICO_INTERNAL_ERROR_FIRMWARE_NULL", "PICO_FIRMWARE_FAILED_TO_BE_CHANGED", "PICO_FIRMWARE_FAILED_TO_RELOAD", "PICO_FIRMWARE_FAILED_TO_BE_UPDATE", "PICO_FIRMWARE_VERSION_OUT_OF_RANGE", "PICO_NO_APPS_AVAILABLE", "PICO_UNSUPPORTED_APP", "PICO_ADC_POWERED_DOWN\r\nthe adc is powered down when trying to capture data", "PICO_WATCHDOGTIMER\r\nAn internal error has occurred and a watchdog timer has been called.", "PICO_IPP_NOT_FOUND\r\nThe picoipp.dll has not been found.", "PICO_IPP_NO_FUNCTION\r\nA function in the picoipp.dll does not exist.", "PICO_IPP_ERROR\r\nThe Pico IPP call has failed.", "PICO_SHADOW_CAL_NOT_AVAILABLE\r\nShadow calibration is not available on this device.", "PICO_SHADOW_CAL_DISABLED\r\nShadow calibration is currently disabled.", "PICO_SHADOW_CAL_ERROR\r\nShadow calibration error has occurred.", "PICO_SHADOW_CAL_CORRUPT\r\nThe shadow calibration is corrupt.", "PICO_DEVICE_MEMORY_OVERFLOW\r\nThe memory on board the device has overflowed.", "PICO_ADC_TEST_FAILURE\r\nThe device Adc test failed.", "PICO_RESERVED_1", "PICO_SOURCE_NOT_READY\r\nThe PicoSource device is not ready to accept instructions.", "PICO_SOURCE_INVALID_BAUD_RATE", "PICO_SOURCE_NOT_OPENED_FOR_WRITE", "PICO_SOURCE_FAILED_TO_WRITE_DEVICE", "PICO_SOURCE_EEPROM_FAIL", "PICO_SOURCE_EEPROM_NOT_PRESENT", "PICO_SOURCE_EEPROM_NOT_PROGRAMMED", "PICO_SOURCE_LIST_NOT_READY", "PICO_SOURCE_FTD2XX_NOT_FOUND", "PICO_SOURCE_FTD2XX_NO_FUNCTION"] ("PICO_STATUS strings")
  # "Subtract 5000 offset from legacy PICO_STATUS code"
  # "Adding 5000 offset to support legacy code"
  # "From PicoStatus.h"
  n1 = Array Size(array=w1) -> (size(s)=w7:i32)
  n2 = for {
    N: w7 -> [_]
    tunnel: w1 -> [w10] mode=indexing
    tunnel: [w11] -> w6 mode=indexing
    n3 = Add(x=w10, y=u32 5000) -> (x+y=w11:u32)
  }
  "[user-defined codes]" <- w6
  n4 = Unbundle By Name("error in") -> ("code"=w5:i32)  [unwired: 2 out]
  n5 = Subtract(x=w5, y=5000) -> (x-y=w4:i32)
  n6 = case shown="Default" w4 {
    selector: w4 -> [w17 _]
    tunnel: w2 -> [w20 _]
    tunnel: w1 -> [w19 _]
    tunnel: [w18 "PICO_STATUS OK " ("string")] -> w8
    frame Default {
      n7 = Search 1D Array(1D array=w19, element=w17) -> (index of element=w15:i32)  [unwired: 1 in]
      n8 = Number To Decimal String(number=w17) -> (decimal integer string=w13:string)  [unwired: 1 in]
      n9 = Equal?(x=w15, y=-1) -> (x = y?=w16:bool)
      n10 = case shown="True" w16 {
        tunnel: w20 -> [w27 _]
        tunnel: w15 -> [w26 _]
        tunnel: [w24 w31] -> w18
        tunnel: w13 -> [w21 w28]
        frame False {
          n11 = Index Array(array=w27, index=w26) -> (element=w25:string)
          n12 = Concatenate Strings(w25, "\r", "Error code " ("string"), w21) -> (w24:string)
        }
        frame True {
          n13 = Concatenate Strings("PICO_STATUS Unknown Error " ("string"), "\r", "Error code " ("string"), w28) -> (w31:string)
        }
      }
    }
    frame 0 {
    }
  }
  "String" <- w8
  "[user-defined descriptions]" <- w2
